vi "Serialize - JSON.vi"(8 "error in":errorcluster, 11 "Vaisala Data in":refnum<class "Vaisala Data.lvclass">) -> (0 "error out":errorcluster, 2 "Serialized JSON":string, 3 "Vaisala Data out":refnum<class "Vaisala Data.lvclass">)   [LabVIEW 2015, in "Vaisala Library.lvlib" / "Vaisala Data.lvclass"]
uses:
  Vaisala Data.lvclass
  <vilib>/MSR Consulting, LLC/General Reuse/Data/Data.lvclass/Data.ctl
  Vaisala Data.lvclass/Vaisala Data.ctl
  <vilib>/MSR Consulting, LLC/General Reuse/Data/Read Data ID.vi
  <vilib>/MSR Consulting, LLC/General Reuse/Data/Data.lvclass
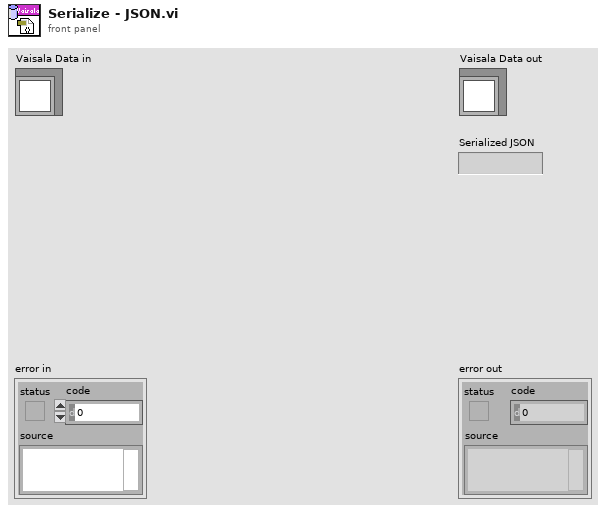
[diagram p1: front panel]
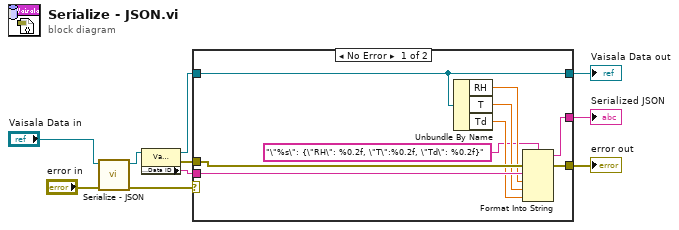
[diagram p0: block diagram]
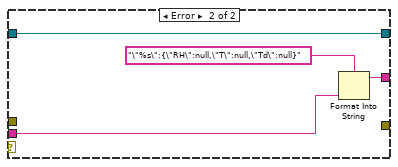
[diagram p2: hidden frame]
diagram:
  n1 = call-parent "Serialize - JSON.vi"("error in"="error in", "Data in"="Vaisala Data in") -> ("error out"=w2:errorcluster, "Data out"=w5:refnum<class "Vaisala Data.lvclass">)  [unwired: 7 in, 1 out]
  n2 = property class="Vaisala Data"(reference=w5) -> (reference out=w3:refnum<class "Vaisala Data.lvclass">, error out=w9:errorcluster, "Accessors:Data ID"=w10:string)  [unwired: 1 in]
  n3 = case shown="No Error" w2 {
    tunnel: w10 -> [w19 w22]
    tunnel: w9 -> [w18 _]
    tunnel: [w17 _] -> w8
    tunnel: [w16 w20] -> w7
    tunnel: w3 -> [w11 w21]
    tunnel: [w11 w21] -> w1
    frame No Error {
      n4 = Unbundle By Name(w11) -> ("RH"=w15:dbl, "T"=w14:dbl, "Td"=w13:dbl)
      n5 = Format Into String(format string="\"%s\": {\"RH\": %0.2f, \"T\":%0.2f, \"Td\": %0.2f}", error in=w18, w19, w15, w14, w13) -> (resulting string=w16:string, error out=w17:errorcluster)  [unwired: 1 in]
    }
    frame Error {
      n6 = Format Into String(format string="\"%s\":{\"RH\":null,\"T\":null,\"Td\":null}", w22) -> (resulting string=w20:string)  [unwired: 2 in, 1 out]
    }
  }
  "error out" <- w8
  "Vaisala Data out" <- w1
  "Serialized JSON" <- w7
